vi "Check Abort or Pause Message During Execution Task.vi"(8 "error in (no error)":errorcluster, 11 "System Actor in":refnum<class "System Actor.lvclass">) -> (0 "error out":errorcluster, 1 "CMD":T1 caption="Enum 3", 2 "Abort?":bool, 3 "System Actor out":refnum<class "System Actor.lvclass">, 4 "Message Out":refnum<class "Message.lvclass">)   [LabVIEW 2024, in "System Actor.lvclass"]
uses:
  System Actor.lvclass
  Message/Type Def/General CMD.ctl
  Message/Message.lvclass
  Message/Message.lvclass/Message.ctl
  Message/Public Data/Read CMD Type.vi
  Message/Public Data/Read General CMD.vi
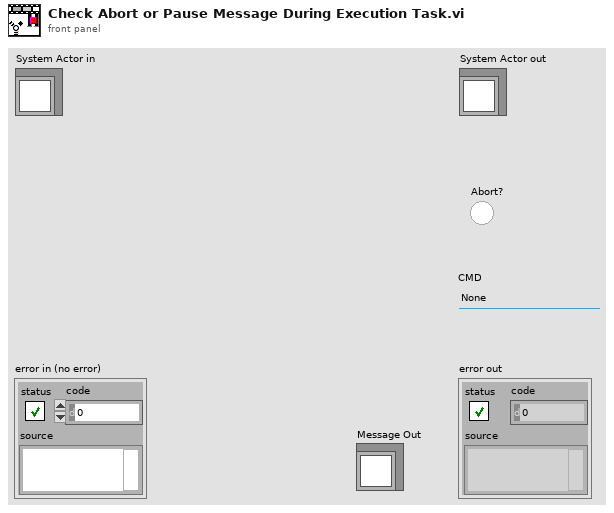
[diagram p1: front panel]
types:
  T1 = typedef "General CMD.ctl" = enum16{"None", "Stop", "Abort", "Running Task", "Running Batch Tasks", "Task Self Running", "Emergency Stop", "Subscribe", "UnSubscribe", "Pause", "Receive Parameters", "Active", "Resume"}
  T2 = typedef "CMD Type.ctl" = enum16{"None", "General CMD", "1st CMD", "2nd CMD", "3rd CMD", "4th CMD", "5th CMD", "6th CMD", "7th CMD"}
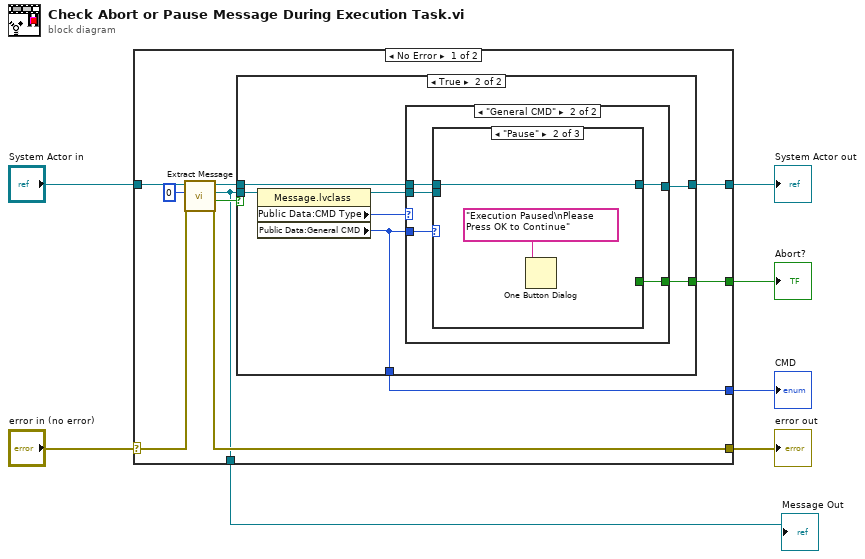
[diagram p0: block diagram]
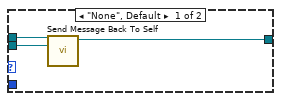
[diagram p3: hidden frame]
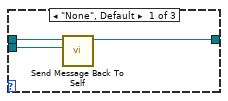
[diagram p4: hidden frame]
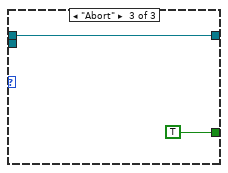
[diagram p5: hidden frame]
diagram:
  n1 = case shown="No Error" "error in (no error)" {
    selector: "error in (no error)" -> [w15 w42]
    tunnel: [w14 w42] -> w6
    tunnel: [w11 w41] -> w4
    tunnel: "System Actor in" -> [w17 w41]
    tunnel: [w10 _] -> w3
    tunnel: [w9 _] -> w2
    tunnel: [w8 _] -> w1
    frame No Error {
      n2 = call-dynamic "Extract Message.vi"("error in (no error)"=w15, "Wait"=0, "System Actor in"=w17) -> ("error out"=w14:errorcluster, "Valid"=w13:bool, "Message Out"=w8:refnum<class "Message.lvclass">, "System Actor out"=w12:refnum<class "System Actor.lvclass">)  [unwired: 5 in]
      n3 = case shown="True" w13 {
        tunnel: w12 -> [w18 w22]
        tunnel: [w18 w21] -> w11
        tunnel: w8 -> [_ w25]
        tunnel: [_ w20] -> w10
        tunnel: [_ w19] -> w9
        frame False {
        }
        frame True {
          n4 = property class="Message.lvclass"(reference=w25) -> (reference out=w23:refnum<class "Message.lvclass">, "Public Data:CMD Type"=w24:T2, "Public Data:General CMD"=w19:T1)  [unwired: 1 in, 1 out]
          n5 = case shown="\"General CMD\"" w24 {
            tunnel: w23 -> [w27 w30]
            tunnel: w22 -> [w28 w32]
            tunnel: [w26 w31] -> w21
            tunnel: w19 -> [_ w33]
            tunnel: [_ w29] -> w20
            frame "None", Default {
              n6 = call "Send Message Back To Self.vi"("Message In"=w27, "System Actor in"=w28) -> ("System Actor out"=w26:refnum<class "System Actor.lvclass">)  [unwired: 8 in, 1 out]
            }
            frame "General CMD" {
              n7 = case shown="\"Pause\"" w33 {
                tunnel: w32 -> [w36 w38 w40]
                tunnel: [w35 w38 w40] -> w31
                tunnel: w30 -> [w34 _ _]
                tunnel: [_ _ TRUE ("Abort?")] -> w29
                frame "None", Default {
                  n8 = call "Send Message Back To Self.vi"("Message In"=w34, "System Actor in"=w36) -> ("System Actor out"=w35:refnum<class "System Actor.lvclass">)  [unwired: 8 in, 1 out]
                }
                frame "Pause" {
                  n9 = One Button Dialog(message="Execution Paused\nPlease Press OK to Continue") -> ()  [unwired: 1 in, 1 out]
                }
                frame "Abort" {
                }
              }
            }
          }
        }
      }
    }
    frame Error {
    }
  }
  "error out" <- w6
  "System Actor out" <- w4
  "Abort?" <- w3
  "CMD" <- w2
  "Message Out" <- w1
